vi "Launch Keypad Dialog Box.vi"(4 "Auto-stop? (T)":bool=TRUE, 8 "error in (no error)":errorcluster, 9 "Parameter Name":string, 10 "Reply Transport":refnum<class "ITransport.lvclass">, 11 "Dialog Launcher In":refnum<class "IViewable.lvclass">) -> (0 "error out":errorcluster, 3 "Dialog Launcher Out":refnum<class "IViewable.lvclass">)   [LabVIEW 2017, in "KeypadDialogBox.lvlib" / "KeypadDialogBox.lvclass"]
uses:
  KeypadDialogBox.lvclass
  gpm_packages/@cs/mva-viewable/Source/IViewable/IViewable/IViewable.lvclass
  C:/Program Files (x86)/National Instruments/LabVIEW 2017/vi.lib/ActorFramework/Actor/Actor.lvclass
  gpm_packages/@cs/transport/Source/ITransport/ITransport.lvclass
  KeypadDialogBox.lvclass/KeypadDialogBox.ctl
  <vilib>/ActorFramework/Actor/Actor.lvclass
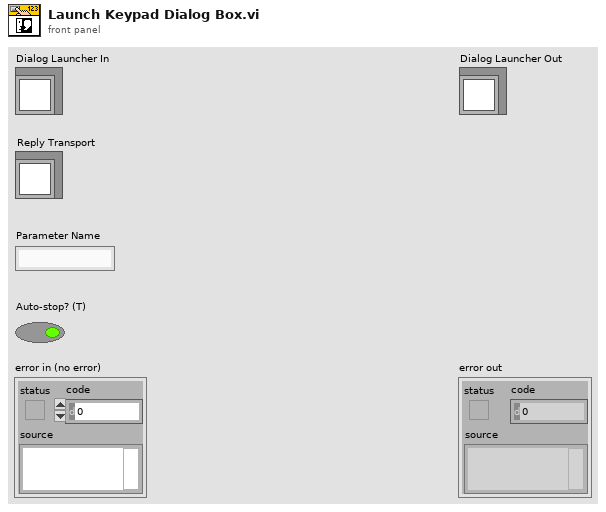
[diagram p1: front panel]
types:
  T1 = enum32{"Invalid", "Default", "Floating", "Floating/Auto-Hide", "Modal"}
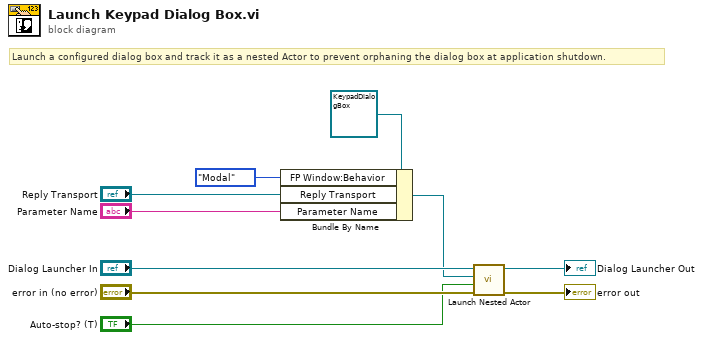
[diagram p0: block diagram]
diagram:
  # "Launch a configured dialog box and track it as a nested Actor to prevent orphaning the dialog box at application shutdown."
  n1 = Bundle By Name(cluster=refnum<class "KeypadDialogBox.lvclass"> refnum ("OneButtonDialogBox in"), "FP Window:Behavior"=T1."Modal", "Reply Transport"="Reply Transport", "Parameter Name"="Parameter Name") -> (w3:refnum<class "KeypadDialogBox.lvclass">)
  n2 = call <vilib>:"Launch Nested Actor.vi"("error in (no error)"="error in (no error)", "Auto-stop? (T)"="Auto-stop? (T)", "Nested Actor"=w3, "Caller Actor in"="Dialog Launcher In") -> ("error out"=→"error out":errorcluster, "Caller Actor out"=→"Dialog Launcher Out":refnum<class "IViewable.lvclass">)  [unwired: 5 in, 1 out]
